vi "SICK VISA Init.vi"() -> ()   [LabVIEW 2009]
uses:
  <vilib>/Instr/_visa.llb/VISA Configure Serial Port (Instr).vi
panel:
  out "Equal Responses":bool[](array[boolean])
  out "Numeric":i32
  out "Expected Responses":string[](array[string])
  out "Actual Responses":string[](array[string])
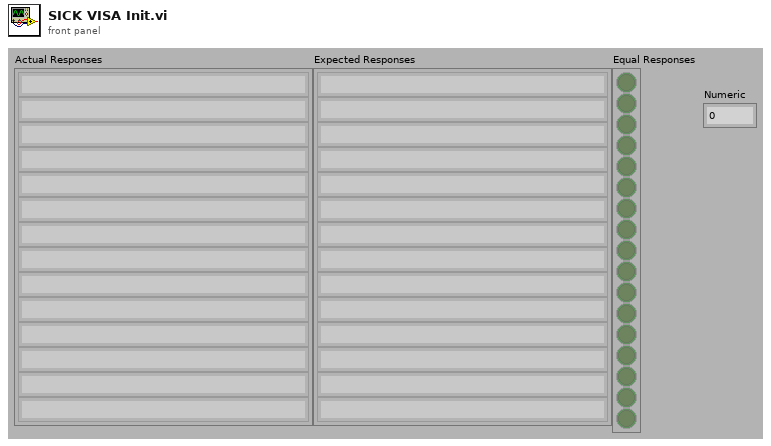
[diagram p1: front panel]
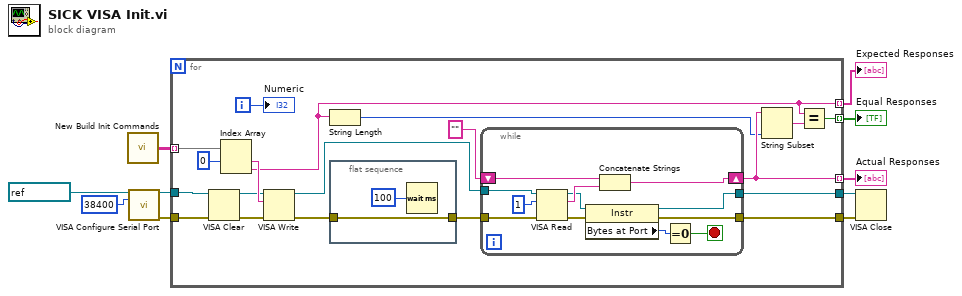
[diagram p0: block diagram]
diagram:
  n1 = call "New Build Init Commands.vi"() -> ("SICK Commands"=w4:string[][])
  n2 = call-poly "VISA Configure Serial Port"("VISA resource name"=refnum<visa-resource-name> "COM1", "baud rate (9600)"=u32 38400) -> ("VISA resource name out"=w10:refnum<visa-resource-name>, "error out"=w9:errorcluster)  [unwired: 12 in]
  n3 = for {
    tunnel: w10 -> [w21]
    tunnel: w9 -> [w22]
    tunnel: [w29] -> w6
    tunnel: [w28] -> w5
    tunnel: w4 -> [w11] mode=indexing
    tunnel: [w16] -> w3 mode=indexing
    tunnel: [w14] -> w2 mode=indexing
    tunnel: [w12] -> w1 mode=indexing
    i -> [w19]
    n4 = VISA Clear(VISA resource name=w21, error in (no error)=w22) -> (VISA resource name out=w24:refnum<visa-resource-name>, error out=w23:errorcluster)
    n5 = Index Array(array=w11, index #1=0 ("index")) -> (element #1=w26:string, element #2=w14:string)  [unwired: 1 in]
    n6 = VISA Write(VISA resource name=w24, write buffer=w26, error in (no error)=w23) -> (VISA resource name out=w20:refnum<visa-resource-name>, error out=w17:errorcluster)  [unwired: 1 out]
    n7 = String Length(string=w14) -> (length=w15:i32)
    n8 = flat-sequence {
      tunnel: [w31] -> w18
      tunnel: w17 -> [w31]
      frame #0 {
        n9 = Wait (ms)(milliseconds to wait=u32 100) -> ()  [unwired: 1 out]
      }
    }
    n10 = while {
      tunnel: [w33] -> w29
      tunnel: [w32] -> w28
      tunnel: w20 -> [w43]
      tunnel: w18 -> [w42]
      shift-right: [w40] -> w16
      shift-left: "" -> [w39]
      stop <- w35 stop-if-true
      n11 = VISA Read(VISA resource name=w43, byte count=u32 1, error in (no error)=w42) -> (VISA resource name out=w37:refnum<visa-resource-name>, read buffer=w41:string, error out=w36:errorcluster)  [unwired: 1 out]
      n12 = property class="Instr"(reference=w37, error in=w36) -> (reference out=w33:refnum<visa-resource-name>, error out=w32:errorcluster, "Bytes at Port"=w34:u32)
      n13 = Concatenate Strings(w39, w41) -> (w40:string)
      n14 = Equal To 0?(x=w34) -> (x = 0?=w35:bool)
    }
    n15 = String Subset(string=w16, length (rest)=w15) -> (substring=w13:string)  [unwired: 1 in]
    n16 = Equal?(x=w14, y=w13) -> (x = y?=w12:bool)
    "Numeric" <- w19
  }
  "Actual Responses" <- w3
  "Expected Responses" <- w2
  "Equal Responses" <- w1
  n17 = VISA Close(VISA resource name=w6, error in (no error)=w5) -> ()  [unwired: 1 out]
